vi "Helm Calculate Throttle Values Test.vi"(8 "error in (no error)":errorcluster) -> (0 "error out":errorcluster)   [LabVIEW 2015]
panel:
  out "Ts":i16
  out "Tp":i16
  in  "R":dbl(slide) scale=-100.0..100.0
  in  "T":dbl(slide) scale=-2000.0..2000.0
  out "TS":dbl(slide) scale=-1000.0..1000.0
  out "PT":dbl(slide) scale=-1000.0..1000.0
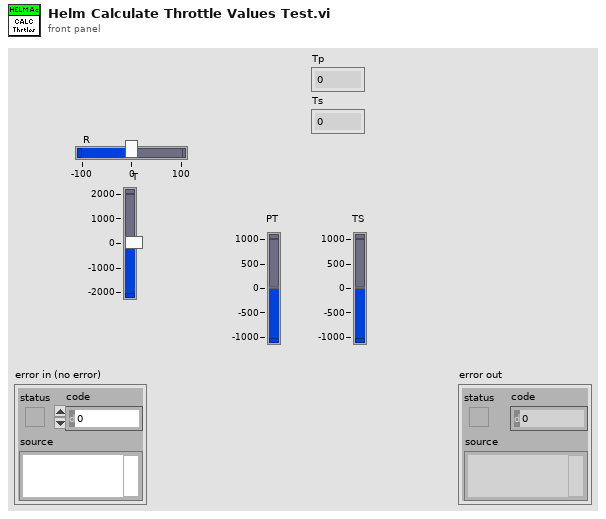
[diagram p1: front panel]
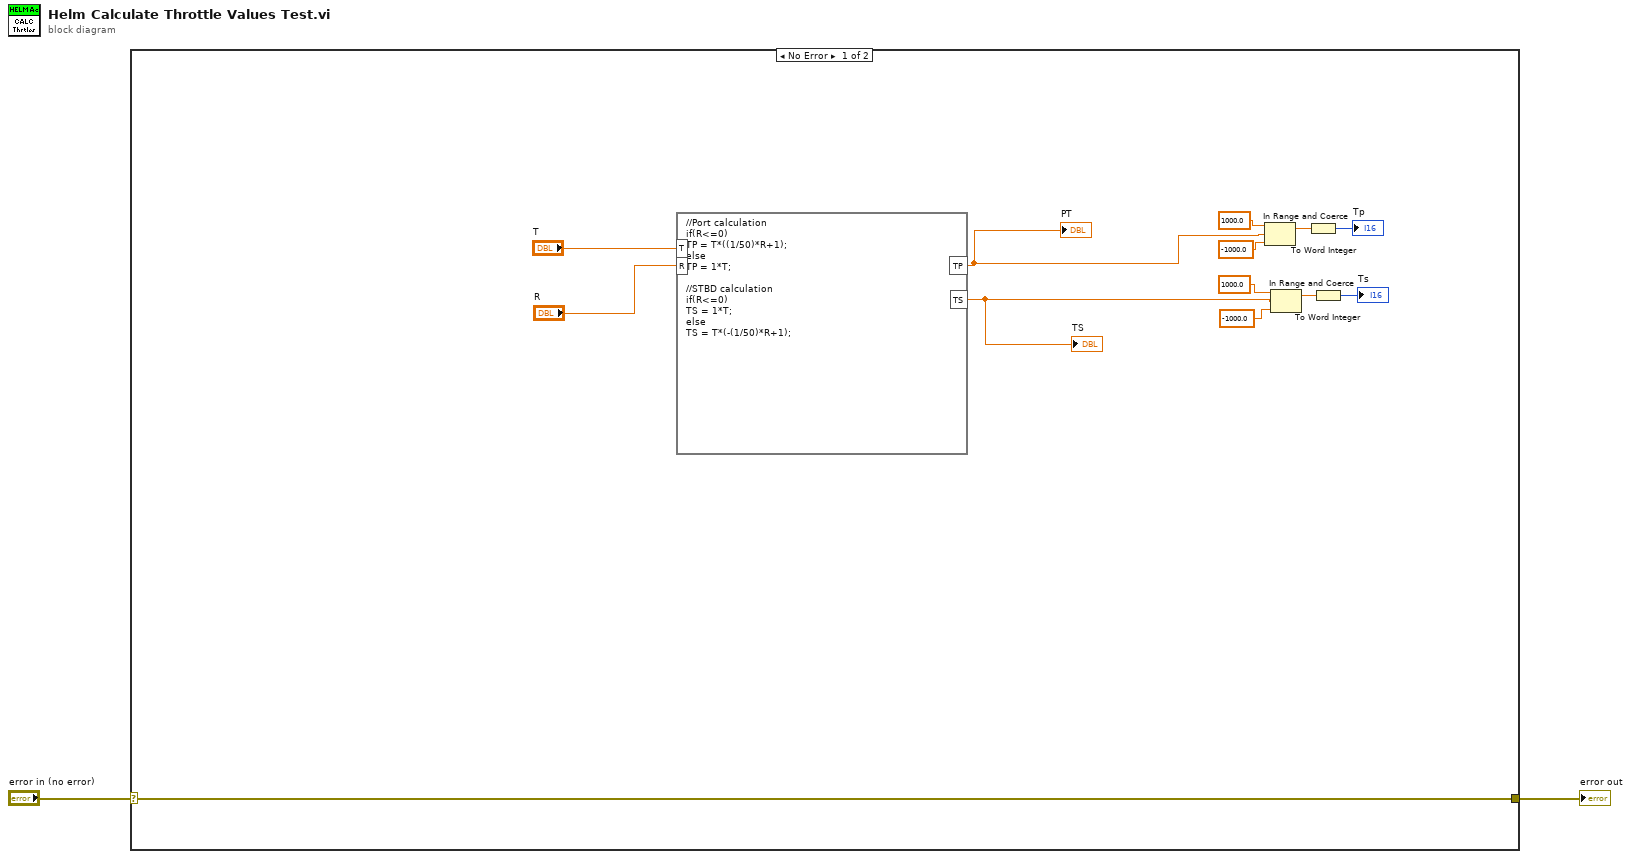
[diagram p0: block diagram]
diagram:
  n1 = case shown="No Error" "error in (no error)" {
    selector: "error in (no error)" -> [w15 w16]
    tunnel: [w15 w16] -> w1
    frame No Error {
      n2 = formula code="//Port calculation\nif(R<=0)\nTP = T*((1/50)*R+1);\nelse\nTP = 1*T;\n\n//STBD calculation\nif(R<=0)\nTS = 1*T;\nelse\nTS = T*(-(1/50)*R+1);"("R"="R", "T"="T") -> ("TP"=w6:dbl, "TS"=w5:dbl)
      "PT" <- w6
      "TS" <- w5
      n3 = In Range and Coerce(upper limit=1000.0, x=w6, lower limit=-1000.0) -> (coerced(x)=w8:dbl)  [unwired: 1 out]
      n4 = In Range and Coerce(upper limit=1000.0, x=w5, lower limit=-1000.0) -> (coerced(x)=w7:dbl)  [unwired: 1 out]
      n5 = To Word Integer(number=w8) -> (16bit integer=→"Tp":i16)
      n6 = To Word Integer(number=w7) -> (16bit integer=→"Ts":i16)
    }
    frame Error {
    }
  }
  "error out" <- w1
